vi "DMM Wrapper.vi"(7 "Control":T1=enum."Read", 8 "error in":errorcluster, 10 "Setting":T2={"Resolution (Digits)"=5.5, "Current Source (Amps)"=0.001, "Range"=2.0, "Measurement Type"=enum."DC Volts"} {"Range" format="%.2p"; "Current Source (Amps)" items=["1uA"=1e-06, "10uA"=1e-05, "100uA"=0.0001, "1mA"=0.001]; "Resolution (Digits)" items=["3 1/2"=3.5, "4 1/2"=4.5, "5 1/2"=5.5, "6 1/2"=6.5, "7 1/2"=7.5]}, 11 "Alias name":string="DUT0_Volt_rail") -> (0 "error out":errorcluster={"status"=TRUE, "code"=-1074130544, "source"="niSwitch Connect Channels (Multiple).vi<ERR>IVI: (Hex 0xBFFA1190) The session handle is not valid.\n\n "}, 3 "Measurement":dbl=7.565564780388918)   [LabVIEW 2021, in "MIO Wrappers.lvlib"]
uses:
  MIO Wrappers.lvlib
  Controls/DMM States.ctl
  Load INI/Controls/Instruments_Data.ctl
  Load INI/Controls/MUX_Data.ctl
  Load INI/Controls/DMM_Data.ctl
  <instrlib>/niDMM/nidmm.llb/niDMM Configure Measurement Digits.vi
  <instrlib>/niSwitch/niSwitch.llb/niSwitch Connect Channels (Multiple).vi
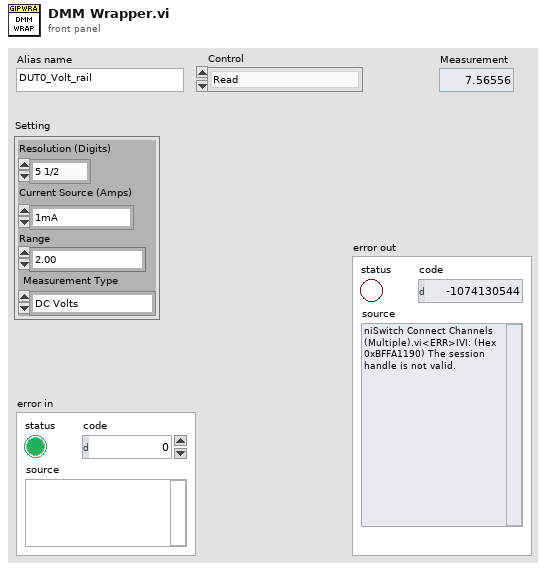
[diagram p1: front panel]
types:
  T1 = typedef "MIO Wrappers.lvlib/DMM States.ctl" = enum16{"Init", "Get Switch Ref", "Config", "Read", "Close"}
  T2 = cluster{"Resolution (Digits)":dbl, "Current Source (Amps)":dbl, "Range":dbl, "Measurement Type":enum16{"DC Volts", "AC Volts", "DC Current", "AC Current", "2-wire Resistance", "4-wire Resistance", "Diode", "Frequency", "Period", "AC Volts DC Coupled", "Capacitance", "Inductance", "Temperature"}}
  T3 = typedef "Instruments_Data.ctl" = cluster{"Alias":string, "Resource ":string}
  T4 = cluster{"DMM ref":refnum<k15>, "SW Refs":refnum<k15>[]}
  T5 = typedef "MUX_Data.ctl" = cluster{"Alias":string, "Topology":string}
  T6 = typedef "DMM_Data.ctl" = cluster{"Alias":string, "MUX":string, "Route":string}
  T7 = enum16{"DC Volts", "AC Volts", "DC Current", "AC Current", "2-wire Resistance", "4-wire Resistance", "Diode", "Frequency", "Period", "AC Volts DC Coupled", "Capacitance", "Inductance", "Temperature"}
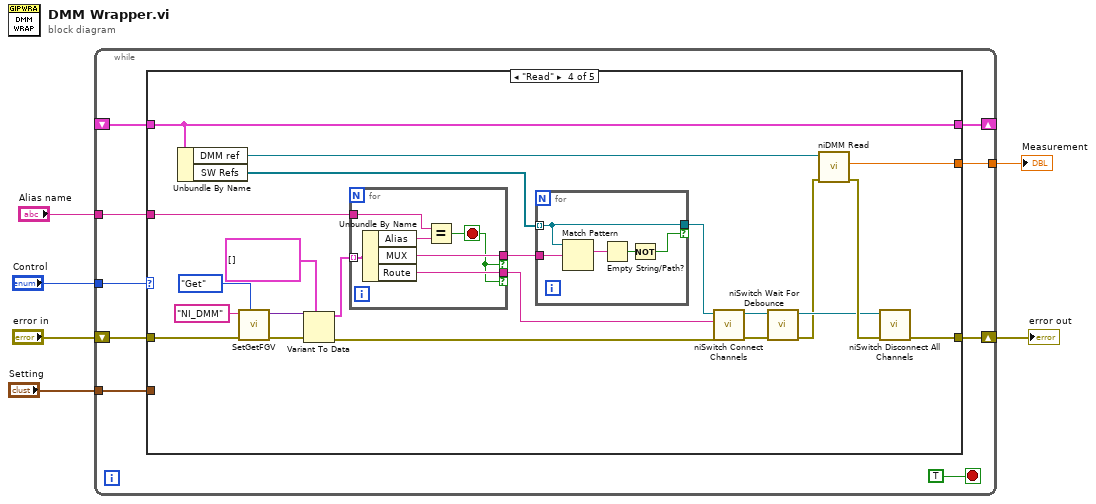
[diagram p0: block diagram]
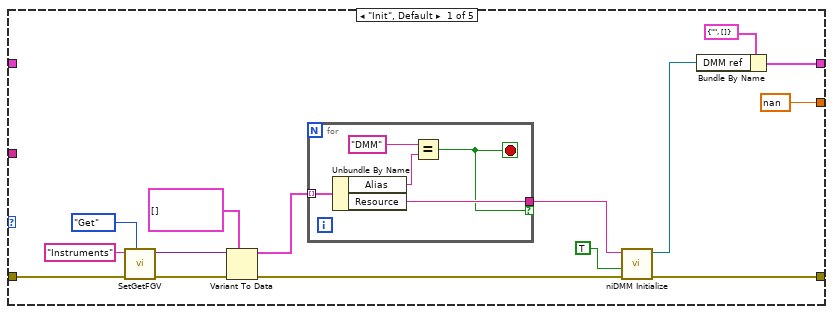
[diagram p2: hidden frame]
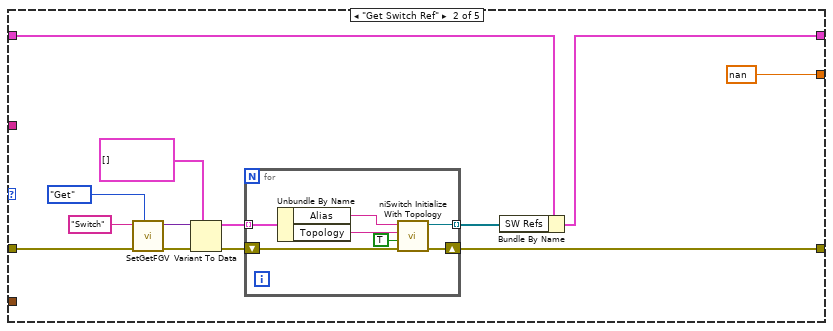
[diagram p3: hidden frame]
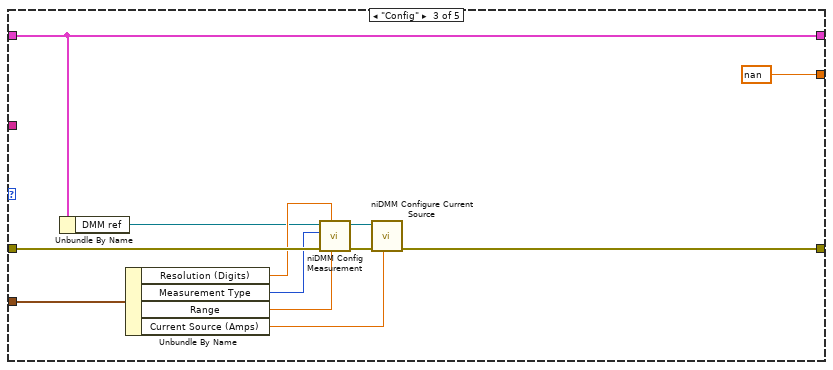
[diagram p4: hidden frame]
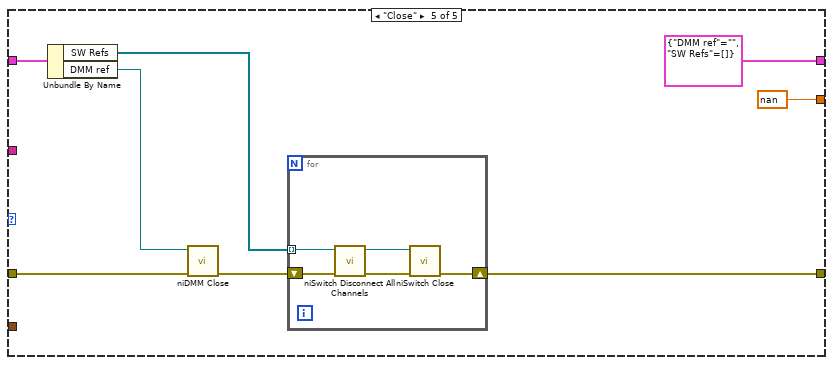
[diagram p5: hidden frame]
diagram:
  n1 = while {
    tunnel: "Setting" -> [w13]
    tunnel: [w12] -> w5
    tunnel: "Control" -> [w11]
    shift-right: [w14] -> w2
    shift-left: "error in" -> [w15]
    shift-right: [w9] -> _
    shift-left: _ -> [w8]
    tunnel: "Alias name" -> [w7]
    stop <- TRUE stop-if-true
    n2 = case shown="\"Read\"" w11 {
      tunnel: w15 -> [w24 w40 w66 w86 w104]
      tunnel: [w27 w39 w57 w88 w103] -> w14
      tunnel: [w29 w37 w58 w89 T4 {"DMM ref"="", "SW Refs"=[]}] -> w9
      tunnel: w8 -> [_ w38 w58 w89 w105]
      tunnel: w13 -> [_ _ w64 _ _]
      tunnel: [nan nan nan w87 nan] -> w12
      tunnel: w7 -> [_ _ _ w68 _]
      frame "Init", Default {
        n3 = call "SetGetFGV.vi"("Method (Get)"=enum16{"Get", "Set"}."Get", "error in"=w24, "FGVname"="Instruments" ("Name")) -> ("error out"=w23:errorcluster, "Data out"=w19:variant)  [unwired: 7 in]
        n4 = Variant To Data(error in=w23, type=T3[] [], Variant=w19) -> (data=w17:T3[], error out=w20:errorcluster)
        n5 = for {
          tunnel: w17 -> [w35] mode=indexing
          tunnel: [w32] -> w16 if=w31
          stop <- w31 stop-if-true
          n6 = Unbundle By Name(w35) -> ("Alias"=w34:string, "Resource"=w32:string)
          n7 = Equal?(x="DMM" ("Name"), y=w34) -> (x = y?=w31:bool)
        }
        n8 = call <instrlib>:"niDMM Initialize.vi"("error in (no error)"=w20, "Reset"=TRUE ("ID Query? (T: Yes)"), "Instrument Descriptor"=w16) -> ("error out"=w27:errorcluster, "instrument handle out"=w25:refnum<k15>)  [unwired: 1 in, 6 out]
        n9 = Bundle By Name(cluster=T4 {"DMM ref"="", "SW Refs"=[]}, "DMM ref"=w25) -> (w29:T4)
      }
      frame "Get Switch Ref" {
        n10 = call "SetGetFGV.vi"("Method (Get)"=enum16{"Get", "Set"}."Get", "error in"=w40, "FGVname"="Switch" ("Name")) -> ("error out"=w48:errorcluster, "Data out"=w47:variant)  [unwired: 7 in]
        n11 = Variant To Data(error in=w48, type=T5[] [], Variant=w47) -> (data=w46:T5[], error out=w45:errorcluster)
        n12 = for {
          tunnel: w46 -> [w54] mode=indexing
          tunnel: [w51] -> w44 mode=indexing
          shift-right: [w50] -> w39
          shift-left: w45 -> [w55]
          n13 = Unbundle By Name(w54) -> ("Alias"=w53:string, "Topology"=w52:string)
          n14 = call <instrlib>:"niSwitch Initialize With Topology.vi"("error in (no error)"=w55, "reset device (boolean value)"=TRUE, "topology name"=w52, "resource name"=w53) -> ("error out"=w50:errorcluster, "instrument handle out"=w51:refnum<k15>)  [unwired: 6 in]
        }
        n15 = Bundle By Name(cluster=w38, "SW Refs"=w44) -> (w37:T4)
      }
      frame "Config" {
        n16 = Unbundle By Name(w58) -> ("DMM ref"=w56:refnum<k15>)
        n17 = Unbundle By Name(w64) -> ("Resolution (Digits)"=w60:dbl, "Measurement Type"=w63:T7, "Range"=w59:dbl, "Current Source (Amps)"=w61:dbl)
        n18 = call-poly <instrlib>:"niDMM Config Measurement.vi"("Range"=w59, "Resolution in Digits"=w60, "error in (no error)"=w66, "Function"=w63, "instrument handle"=w56) -> ("error out"=w67:errorcluster, "instrument handle out"=w65:refnum<k15>)  [unwired: 5 out]
        n19 = call <instrlib>:"niDMM Configure Current Source.vi"("Current Source"=w61, "error in (no error)"=w67, "instrument handle"=w65) -> ("error out"=w57:errorcluster)  [unwired: 1 in, 7 out]
      }
      frame "Read" {
        n20 = Unbundle By Name(w89) -> ("DMM ref"=w72:refnum<k15>, "SW Refs"=w74:refnum<k15>[])
        n21 = call "SetGetFGV.vi"("Method (Get)"=enum16{"Get", "Set"}."Get", "error in"=w86, "FGVname"="NI_DMM" ("Name")) -> ("error out"=w81:errorcluster, "Data out"=w80:variant)  [unwired: 7 in]
        n22 = Variant To Data(error in=w81, type=T6[] [], Variant=w80) -> (data=w71:T6[], error out=w75:errorcluster)
        n23 = for {
          tunnel: [w94] -> w69 if=w92
          tunnel: w71 -> [w95] mode=indexing
          tunnel: [w93] -> w70 if=w92
          tunnel: w68 -> [w91]
          stop <- w92 stop-if-true
          n24 = Unbundle By Name(w95) -> ("Alias"=w90:string, "MUX"=w93:string, "Route"=w94:string)
          n25 = Equal?(x=w91, y=w90) -> (x = y?=w92:bool)
        }
        n26 = for {
          tunnel: w74 -> [w97] mode=indexing
          tunnel: w70 -> [w100]
          tunnel: [w97] -> w73 if=w96
          n27 = Match Pattern(string=w97, regular expression=w100) -> (match substring=w99:string)  [unwired: 1 in, 3 out]
          n28 = Empty String/Path?(string/path=w99) -> (empty?=w98:bool)
          n29 = Not(x=w98) -> (.not. x?=w96:bool)
        }
        n30 = call-poly <instrlib>:"niSwitch Connect Channels.vi"("error in (no error)"=w75, "connection list"=w69, "instrument handle"=w73) -> ("error out"=w76:errorcluster, "instrument handle out"=w83:refnum<k15>)  [unwired: 7 in]
        n31 = call <instrlib>:"niSwitch Wait For Debounce.vi"("error in (no error)"=w76, "instrument handle"=w83) -> ("error out"=w78:errorcluster, "instrument handle out"=w84:refnum<k15>)  [unwired: 1 in, 7 out]
        n32 = call <instrlib>:"niDMM Read.vi"("error in (no error)"=w78, "instrument handle"=w72) -> ("error out"=w85:errorcluster, "Measurement"=w87:dbl)  [unwired: 1 in, 7 out]
        n33 = call <instrlib>:"niSwitch Disconnect All Channels.vi"("error in (no error)"=w85, "instrument handle"=w84) -> ("error out"=w88:errorcluster)  [unwired: 8 in, 1 out]
      }
      frame "Close" {
        n34 = Unbundle By Name(w105) -> ("SW Refs"=w107:refnum<k15>[], "DMM ref"=w101:refnum<k15>)
        n35 = call <instrlib>:"niDMM Close.vi"("error in (no error)"=w104, "instrument handle"=w101) -> ("error out"=w106:errorcluster)  [unwired: 9 in]
        n36 = for {
          tunnel: w107 -> [w109] mode=indexing
          shift-right: [w113] -> w103
          shift-left: w106 -> [w110]
          n37 = call <instrlib>:"niSwitch Disconnect All Channels.vi"("error in (no error)"=w110, "instrument handle"=w109) -> ("error out"=w112:errorcluster, "instrument handle out"=w111:refnum<k15>)  [unwired: 8 in]
          n38 = call <instrlib>:"niSwitch Close.vi"("error in (no error)"=w112, "instrument handle"=w111) -> ("error out"=w113:errorcluster)  [unwired: 9 in]
        }
      }
    }
  }
  "Measurement" <- w5
  "error out" <- w2
